vi "CMD_LOADGEODEF.vi"(6 "Gantry Class in":refnum<class "Gantry Class.lvclass">, 8 "error in (no error)":errorcluster, 10 "Arguments":string[](array[string]), 11 "gScript Interpreter in":refnum<class "gScript Interpreter.lvclass">) -> (0 "error out":errorcluster, 3 "gScript Interpreter out":refnum<class "gScript Interpreter.lvclass">, 4 "Gantry Class out":refnum<class "Gantry Class.lvclass">)   [LabVIEW 2017, in "gScript Interpreter.lvclass"]
uses:
  gScript Interpreter.lvclass
  Shared Components/Gantry Class/Gantry Class.lvclass
  Shared Components/Config Manager Class/Type Definitions/Part Type.ctl
  Shared Components/Config Manager Class/Config Manager Class.lvclass
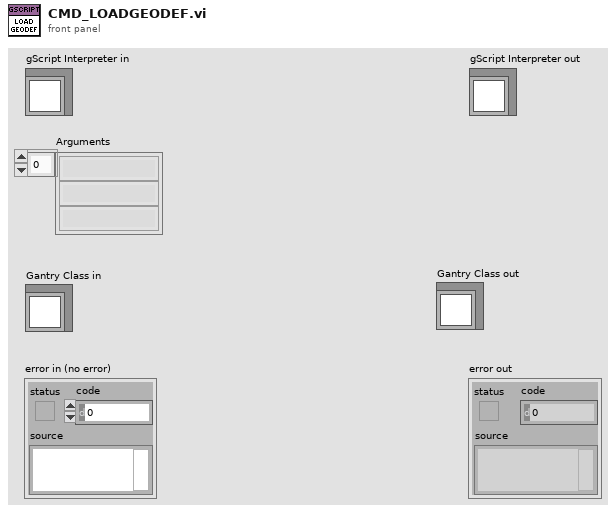
[diagram p1: front panel]
types:
  T1 = typedef "Part Type.ctl" = enum16{"BBM", "HDI", "BARE HDI", "GLUERESERVOIR", "STAMP_1", "STAMP_2", "STAMP_3", "STAMP_4", "STAMP_5", "STAMP_6", "STAMP_7", "STAMP_8", "WEIGHT_1", "WEIGHT_2", "WEIGHT_3", "WEIGHT_4", "WEIGHT_5", "WEIGHT_6", "WEIGHT_7", "WEIGHT_8", "WEIGHT_9", "WEIGHT_10", "WEIGHT_11", "WEIGHT_12", "WEIGHT_13", "WEIGHT_14", "WEIGHT_15", "WEIGHT_16", "PICKER_TOOL", "GRABER_TOOL", "TFPX_HDI_V2"}
  T2 = typedef "Memory Cell.ctl" = cluster{"type":T3, "x":dbl, "y":dbl, "z":dbl, "w":dbl}
  T3 = typedef "Memory Cell Type Enum.ctl" = enum16{"integer", "float", "vector", "rotation"}
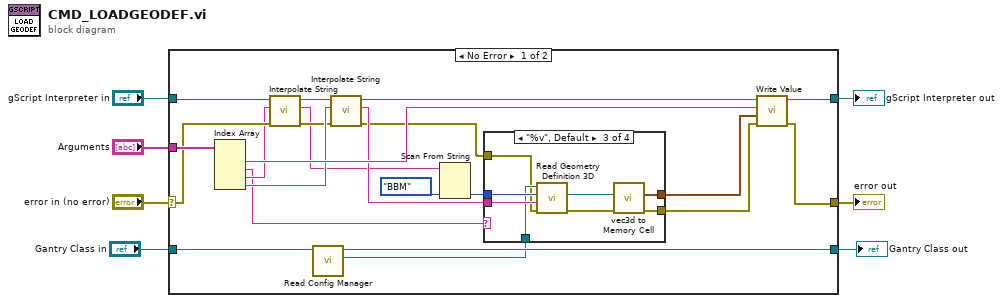
[diagram p0: block diagram]
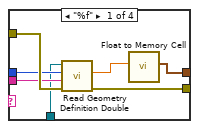
[diagram p2: hidden frame]
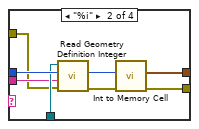
[diagram p3: hidden frame]
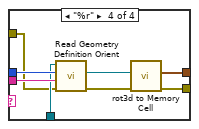
[diagram p4: hidden frame]
diagram:
  n1 = case shown="No Error" "error in (no error)" {
    selector: "error in (no error)" -> [w22 w60]
    tunnel: [w27 w60] -> w6
    tunnel: [w26 w59] -> w4
    tunnel: "gScript Interpreter in" -> [w24 w59]
    tunnel: "Arguments" -> [w28 _]
    tunnel: "Gantry Class in" -> [w25 w58]
    tunnel: [w13 w58] -> w1
    frame No Error {
      n2 = Index Array(array=w28) -> (element #1=w29:string, element #2=w17:string, element #3=w21:string, element #4=w20:string)  [unwired: 4 in]
      n3 = call-dynamic "Interpolate String.vi"("error in (no error)"=w22, "Input String"=w21, "gScript Interpreter in"=w24) -> ("error out"=w19:errorcluster, "Output String"=w15:string, "gScript Interpreter out"=w23:refnum<class "gScript Interpreter.lvclass">)  [unwired: 6 in]
      n4 = call-dynamic "Read Config Manager.vi"("Gantry in"=w25) -> ("Config Manager"=w12:refnum<class "Config Manager Class.lvclass">, "Gantry out"=w13:refnum<class "Gantry Class.lvclass">)  [unwired: 8 in, 1 out]
      n5 = call-dynamic "Interpolate String.vi"("error in (no error)"=w19, "Input String"=w20, "gScript Interpreter in"=w23) -> ("error out"=w11:errorcluster, "Output String"=w18:string, "gScript Interpreter out"=w8:refnum<class "gScript Interpreter.lvclass">)  [unwired: 6 in]
      n6 = Scan From String(input string=w15, default 1=Part_Type."BBM" ("Part Type")) -> (output 1=w14:T1)  [unwired: 3 in, 3 out]
      n7 = case shown="\"%v\", Default" w17 {
        tunnel: w18 -> [w35 w41 w48 w56]
        tunnel: w14 -> [w34 w43 w49 w55]
        tunnel: w12 -> [w33 w42 w47 w54]
        tunnel: w11 -> [w36 w40 w46 w53]
        tunnel: [w30 w39 w50 w57] -> w9
        tunnel: [w31 w37 w44 w51] -> w10
        frame "%f" {
          n8 = call "Read Geometry Definition Double.vi"("error in"=w36, "Feature"=w35, "Part Type"=w34, "Config Manager in"=w33) -> ("error out"=w30:errorcluster, "Geometry Definition"=w32:dbl)  [unwired: 5 in, 1 out]
          n9 = call "Float to Memory Cell.vi"("Float in"=w32) -> ("Memory Cell"=w31:T2)  [unwired: 10 in]
        }
        frame "%i" {
          n10 = call "Read Geometry Definition Integer.vi"("error in"=w40, "Feature"=w41, "Part Type"=w43, "Config Manager in"=w42) -> ("error out"=w39:errorcluster, "Geometry Definition"=w38:i32)  [unwired: 5 in, 1 out]
          n11 = call "Int to Memory Cell.vi"("Numeric"=w38) -> ("Memory Cell"=w37:T2)  [unwired: 10 in]
        }
        frame "%v", Default {
          n12 = call "Read Geometry Definition 3D.vi"("error in"=w46, "Feature"=w48, "Part Type"=w49, "Config Manager in"=w47) -> ("error out"=w50:errorcluster, "Feature Coordinates"=w45:refnum<class "Vec3d Class.lvclass">)  [unwired: 5 in, 1 out]
          n13 = call "vec3d to Memory Cell.vi"("Vec3d in"=w45) -> ("Memory Cell"=w44:T2)  [unwired: 10 in]
        }
        frame "%r" {
          n14 = call "Read Geometry Definition Orient.vi"("error in"=w53, "Feature"=w56, "Part Type"=w55, "Config Manager in"=w54) -> ("error out"=w57:errorcluster, "Orient3d out"=w52:refnum<class "Orient3d Class.lvclass">)  [unwired: 5 in, 1 out]
          n15 = call "rot3d to Memory Cell.vi"("Orient3d in"=w52) -> ("Memory Cell"=w51:T2)  [unwired: 10 in]
        }
      }
      n16 = call-dynamic "Write Value.vi"("error in (no error)"=w9, "Value"=w10, "Address"=w29, "gScript Interpreter in"=w8) -> ("error out"=w27:errorcluster, "gScript Interpreter out"=w26:refnum<class "gScript Interpreter.lvclass">)  [unwired: 6 in]
    }
    frame Error {
    }
  }
  "error out" <- w6
  "gScript Interpreter out" <- w4
  "Gantry Class out" <- w1
